vi "IndexToPoint.vi"(8 "error in (no error)":errorcluster, 9 "column":i32, 10 "row":i32, 11 "Evaluator in":refnum<class "Evaluator.lvclass">) -> (0 "error out":errorcluster, 2 "Point":dbl[](array[numeric]), 3 "Evaluator out":refnum<class "Evaluator.lvclass">)   [LabVIEW 2023, in "Evaluator.lvclass"]
uses:
  Evaluator.lvclass
  Evaluator.lvclass/Evaluator.ctl
  Field_class/Field.lvclass
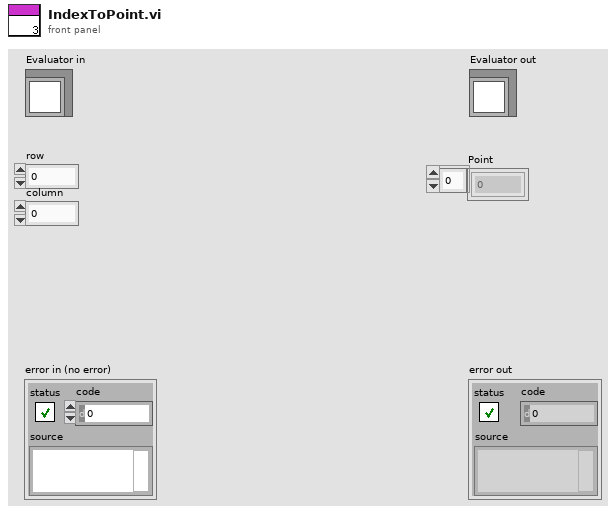
[diagram p1: front panel]
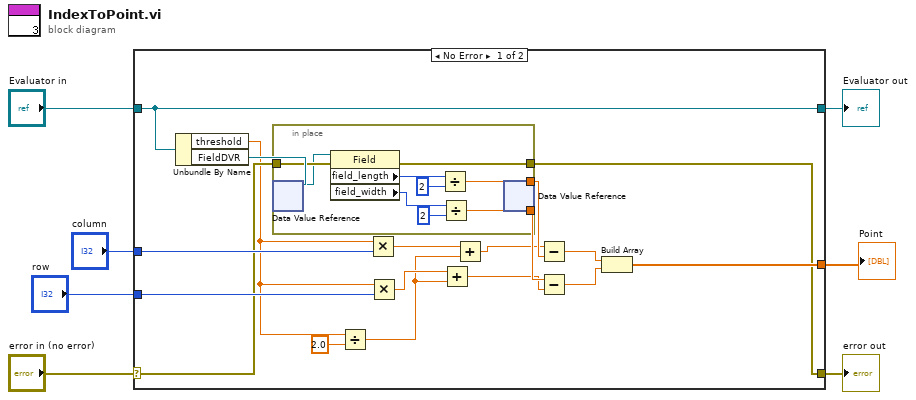
[diagram p0: block diagram]
diagram:
  n1 = case shown="No Error" "error in (no error)" {
    selector: "error in (no error)" -> [w17 w36]
    tunnel: [w16 w36] -> w6
    tunnel: [w25 w35] -> w4
    tunnel: "Evaluator in" -> [w25 w35]
    tunnel: "column" -> [w24 _]
    tunnel: "row" -> [w23 _]
    tunnel: [w18 _] -> w1
    frame No Error {
      n2 = Unbundle By Name(w25) -> ("threshold"=w14:dbl, "FieldDVR"=w15:refnum<data-value>)
      n3 = in-place {
        in-place-border: [w30] -> w22
        in-place-border: [w29] -> w21
        in-place-border: w17 -> [w28]
        in-place-border: [w27] -> w16
        n4 = in-place-dvr #1(w15) -> (w26:refnum<class "Field.lvclass">)  [unwired: 1 out]
        n5 = property class="Field"(reference=w26, error in=w28) -> (error out=w27:errorcluster, "field_length"=w34:i32, "field_width"=w32:i32)  [unwired: 1 out]
        n6 = Divide(x=w34, y=2) -> (x/y=w30:dbl)
        n7 = Divide(x=w32, y=2) -> (x/y=w29:dbl)
        n8 = in-place-dvr #1() -> ()  [unwired: 1 in, 2 out]
      }
      n9 = Divide(x=w14, y=2.0) -> (x/y=w11:dbl)
      n10 = Multiply(x=w14, y=w24) -> (x*y=w10:dbl)
      n11 = Multiply(x=w14, y=w23) -> (x*y=w12:dbl)
      n12 = Add(x=w12, y=w11) -> (x+y=w8:dbl)
      n13 = Add(x=w10, y=w11) -> (x+y=w9:dbl)
      n14 = Subtract(x=w9, y=w22) -> (x-y=w20:dbl)
      n15 = Subtract(x=w21, y=w8) -> (x-y=w19:dbl)
      n16 = Build Array(w20, w19) -> (w18:dbl[])
    }
    frame Error {
    }
  }
  "error out" <- w6
  "Evaluator out" <- w4
  "Point" <- w1
